vi "LoadConfig.vi"(8 "error in":errorcluster, 11 "Global":T1={"Report Folder Path"=path "", "PT1_MIN"=0.0, "PT1_MAX"=0.0, "VENT_PMAX"=0.0, "LOP_TARGET"=0.0, "LOP_RAMP"=0.0, "LOP_LEAK_MAX"=0.0, "HIP_TARGET"=0.0, "HIP_RAMP"=0.0, "HIP_MIN"=0.0, "HIP_MAX"=0.0, "BLEED_TIME"=0.0, "LOP_MAX"=0.0, "LOP_MIN"=0.0, "PT131Com"="COM5", "PT231Com"="COM6", "PT331Com"="COM7", "PT431Com"="COM8", "PT531Com"="COM9", "PT631Com"="COM10"} {"LOP_MIN" format="%#_g PSI"; "LOP_MAX" format="%#_g PSI"; "BLEED_TIME" format="%#_g Sec"; "HIP_MAX" format="%#_g PSI"; "HIP_MIN" format="%#_g PSI"; "HIP_RAMP" format="%#_g Sec"; "HIP_TARGET" format="%#_g PSI"; "LOP_LEAK_MAX" format="%#_g PSI"; "LOP_RAMP" format="%#_g Sec"; "LOP_TARGET" format="%#_g PSI"; "VENT_PMAX" format="%#_g PSI"; "PT1_MAX" format="%#_g PSI"; "PT1_MIN" format="%#_g PSI"}) -> (0 "error out":errorcluster)   [LabVIEW 2018, in "Serial.lvclass"]
uses:
  Serial.lvclass
  Controller/Public Controls/GlobalConfig.ctl
  Queue/Queue Data.ctl
  Queue/State.ctl
  Controller/GUI.lvclass
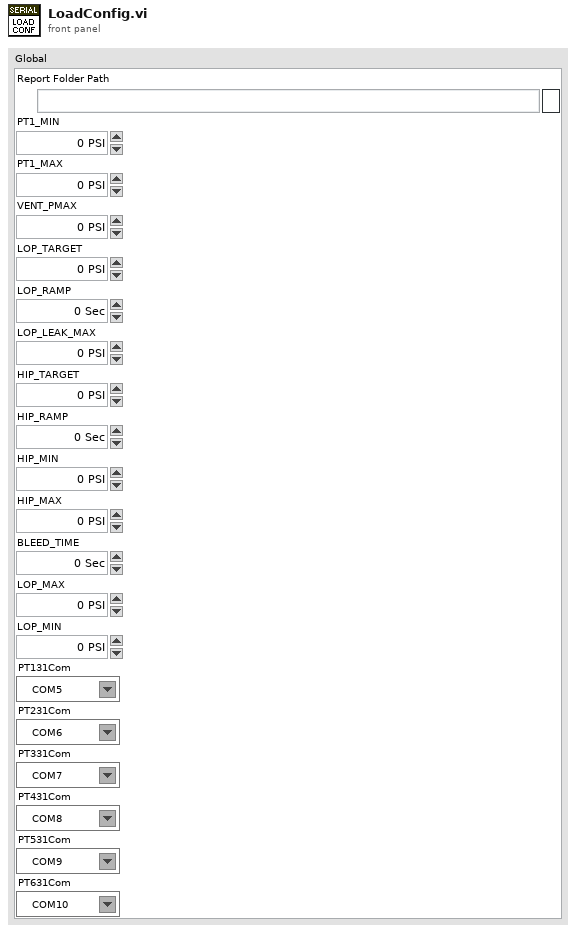
[diagram p1: front panel]
types:
  T1 = typedef "GUI.lvclass/GlobalConfig.ctl" = cluster{"Report Folder Path":path, "PT1_MIN":dbl, "PT1_MAX":dbl, "VENT_PMAX":dbl, "LOP_TARGET":dbl, "LOP_RAMP":dbl, "LOP_LEAK_MAX":dbl, "HIP_TARGET":dbl, "HIP_RAMP":dbl, "HIP_MIN":dbl, "HIP_MAX":dbl, "BLEED_TIME":dbl, "LOP_MAX":dbl, "LOP_MIN":dbl, "PT131Com":refnum<visa-resource-name>, "PT231Com":refnum<visa-resource-name>, "PT331Com":refnum<visa-resource-name>, "PT431Com":refnum<visa-resource-name>, "PT531Com":refnum<visa-resource-name>, "PT631Com":refnum<visa-resource-name>}
  T2 = typedef "Serial.lvclass/Queue Data.ctl" = cluster{"State":T3, "Data":variant}
  T3 = typedef "Serial.lvclass/State.ctl" = enum16{"Initialize", "LoadConfig", "Read", "Error", "Exit"}
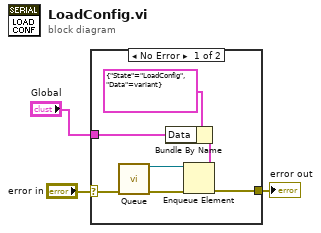
[diagram p0: block diagram]
diagram:
  n1 = case shown="No Error" "error in" {
    selector: "error in" -> [w10 w11]
    tunnel: [w7 w11] -> w3
    tunnel: "Global" -> [w4 _]
    frame No Error {
      n2 = call "Queue.vi"("error in"=w10) -> ("error out"=w9:errorcluster, "queue out"=w8:refnum<queue>)  [unwired: 9 in]
      n3 = Bundle By Name(cluster=T2 {"State"=enum."LoadConfig", "Data"=variant} ("element"), "Data"=w4) -> (w5:T2)
      n4 = Enqueue Element(queue=w8, element=w5, error in (no error)=w9) -> (error out=w7:errorcluster)  [unwired: 1 in, 2 out]
    }
    frame Error {
    }
  }
  "error out" <- w3
